vi "喷码机刷新显示.vi"() -> (2 "刷新显示(16H)":string)   [LabVIEW 2020, in "Untitled Library 1.lvlib"]
uses:
  Untitled Library 1.lvlib
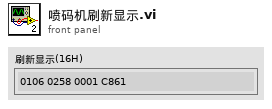
[diagram p1: front panel]
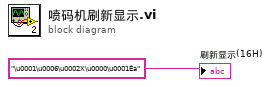
[diagram p0: block diagram]
diagram:
  "刷新显示(16H)" <- "\u0001\u0006\u0002X\u0000\u0001Èa"
